vi "Read Thermocouple Temps.vi"(10 "Thermocouple selector":enum16{"High Accuracy", "High Speed"}(ring)) -> (3 "data":dynamicdata(waveform))   [LabVIEW 2020]
uses:
  <vilib>/DAQmx/configure/timing.llb/DAQmx Timing (Sample Clock).vi
  <resource>/objmgr/daqmx.rc
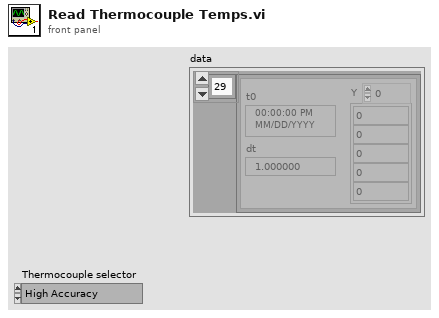
[diagram p1: front panel]
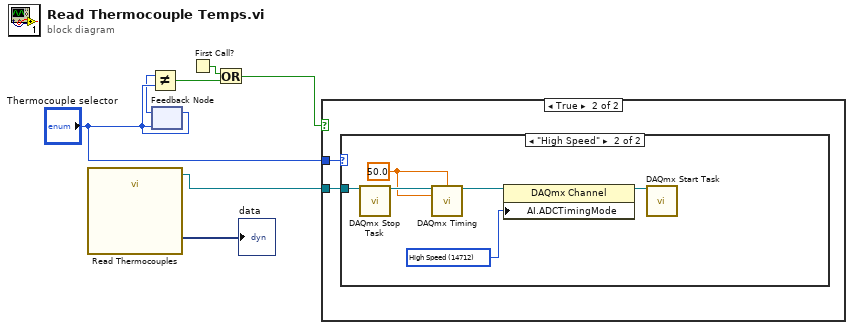
[diagram p0: block diagram]
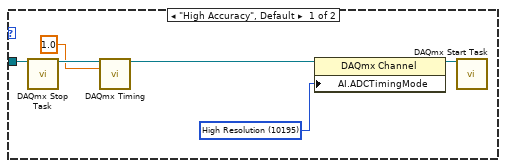
[diagram p3: hidden frame]
diagram:
  n1 = call "Read Thermocouples"() -> ("task out"=w7:refnum<k21>, "data"=→"data":dynamicdata)  [unwired: 16 in, 2 out]
  n2 = feedback-in #1("Thermocouple selector") -> ()
  n3 = feedback #1("Thermocouple selector") -> (w5:enum16{"High Accuracy", "High Speed"})
  n4 = Not Equal?(x=w5, y="Thermocouple selector") -> (x != y?=w2:bool)
  n5 = First Call?() -> (First Call?: T/F=w3:bool)
  n6 = Or(x=w3, y=w2) -> (x .or. y?=w1:bool)
  n7 = case shown="True" w1 {
    tunnel: w7 -> [_ w9]
    tunnel: "Thermocouple selector" -> [_ w8]
    frame False {
    }
    frame True {
      n8 = case shown="\"High Speed\"" w8 {
        tunnel: w9 -> [w13 w20]
        frame "High Accuracy", Default {
          w14 = 10195 items=["Automatic"=16097, "High Resolution"=10195, "High Speed"=14712, "Best 50 Hz Rejection"=14713, "Best 60 Hz Rejection"=14714, "Custom"=10137] ("AI.ADCTimingMode")
          n9 = call <vilib>:"DAQmx Stop Task.vi"("task/channels in"=w13) -> ("task out"=w12:refnum<k21>)  [unwired: 13 in, 1 out]
          n10 = call-poly <vilib>:"DAQmx Timing.vi"("task/channels in"=w12, "rate"=1.0) -> ("task out"=w11:refnum<k21>)  [unwired: 12 in, 1 out]
          n11 = property class="DAQmx Channel"(reference=w11, "AI.ADCTimingMode"=w14) -> (reference out=w15:refnum<k21>)  [unwired: 1 in, 1 out]
          n12 = call <vilib>:"DAQmx Start Task.vi"("task/channels in"=w15) -> ()  [unwired: 13 in, 2 out]
        }
        frame "High Speed" {
          w16 = 50.0 ("rate")
          w19 = 14712 items=["Automatic"=16097, "High Resolution"=10195, "High Speed"=14712, "Best 50 Hz Rejection"=14713, "Best 60 Hz Rejection"=14714, "Custom"=10137] ("AI.ADCTimingMode")
          n13 = call <vilib>:"DAQmx Stop Task.vi"("task/channels in"=w20) -> ("task out"=w18:refnum<k21>)  [unwired: 13 in, 1 out]
          n14 = call-poly <vilib>:"DAQmx Timing.vi"("task/channels in"=w18, "samples per channel"=w16, "rate"=w16) -> ("task out"=w17:refnum<k21>)  [unwired: 11 in, 1 out]
          n15 = property class="DAQmx Channel"(reference=w17, "AI.ADCTimingMode"=w19) -> (reference out=w21:refnum<k21>)  [unwired: 1 in, 1 out]
          n16 = call <vilib>:"DAQmx Start Task.vi"("task/channels in"=w21) -> ()  [unwired: 13 in, 2 out]
        }
      }
    }
  }
